vi "Axis Deadzone.vi"(9 "% Deadzone (Default 5%)":dbl=5.0, 10 "Axis Input":dbl) -> (2 "Output With Deadzone":dbl)   [LabVIEW 2014]
panel:
  # "Puts a deadzone on an axis, making sure that the joystick has to be outside a range to send to a motor.\nDefaults to 5%"
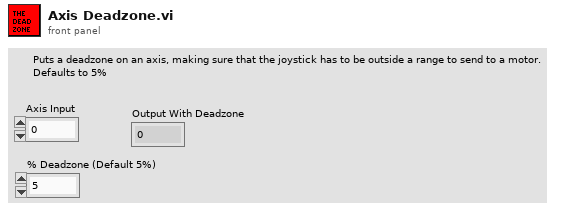
[diagram p1: front panel]
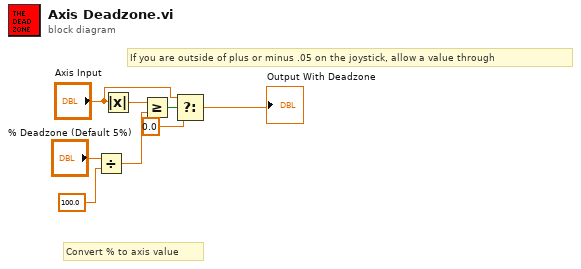
[diagram p0: block diagram]
diagram:
  # "Convert % to axis value"
  # "If you are outside of plus or minus .05 on the joystick, allow a value through"
  n1 = Divide(x="% Deadzone (Default 5%)", y=100.0) -> (x/y=w1:dbl)
  n2 = Absolute Value(x="Axis Input") -> (abs(x)=w8:dbl)
  n3 = Greater Or Equal?(x=w8, y=w1) -> (x >= y?=w7:bool)
  n4 = Select(t="Axis Input", s=w7, f=0.0) -> (s? t:f=→"Output With Deadzone":dbl)
